vi "Plain Text.vi"(7 "Strip Line Ends? (F)":bool, 8 "error in (no error)":errorcluster, 11 "TermBuffer in":refnum<class "TermBuffer.lvclass">) -> (0 "error out":errorcluster, 2 "Contents":string, 3 "TermBuffer out":refnum<class "TermBuffer.lvclass">)   [LabVIEW 2020, in "Terminal.lvlib" / "TermBuffer.lvclass"]
uses:
  TermBuffer.lvclass
  TermBuffer.lvclass/TermBuffer.ctl
  TermLine/TermLine.lvclass
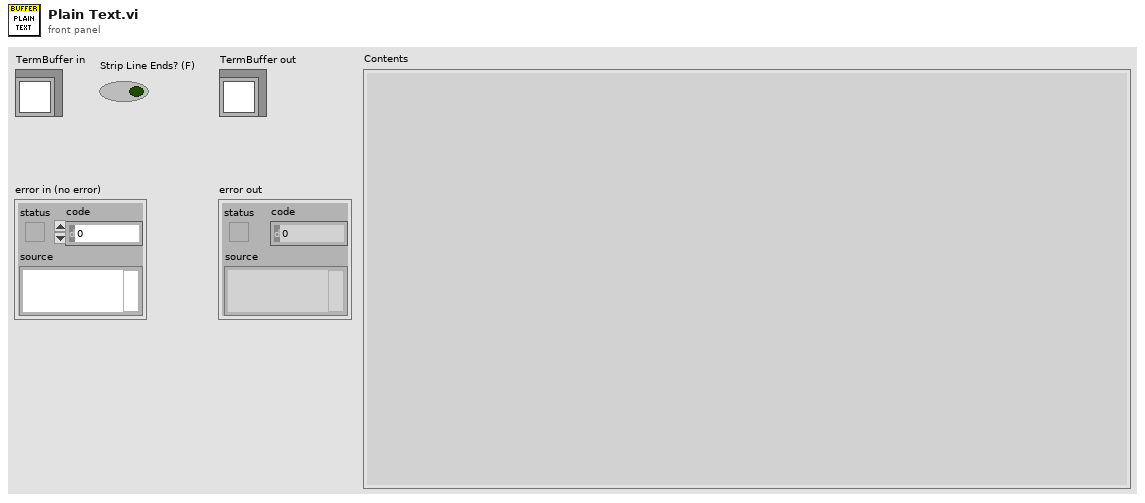
[diagram p1: front panel]
types:
  T1 = typedef "Terminal.lvlib/TermBuffer.lvclass/Ref Data.ctl" = cluster{"Lines":refnum<class "TermLine.lvclass">[], "Rows":i32, "Cols":i32}
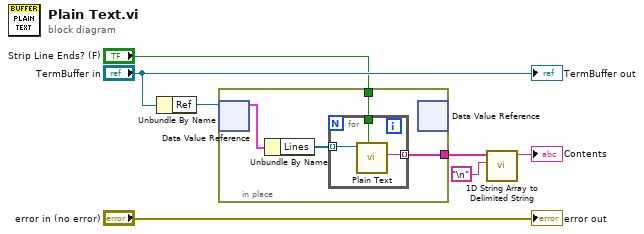
[diagram p0: block diagram]
diagram:
  n1 = Unbundle By Name("TermBuffer in") -> ("Ref"=w6:refnum<data-value>)
  n2 = in-place {
    in-place-border: [w9] -> w4
    in-place-border: "Strip Line Ends? (F)" -> [w8]
    n3 = in-place-dvr #1(w6) -> (w11:T1)  [unwired: 1 out]
    n4 = Unbundle By Name(w11) -> ("Lines"=w10:refnum<class "TermLine.lvclass">[])
    n5 = for {
      tunnel: w10 -> [w14] mode=indexing
      tunnel: [w13] -> w9 mode=indexing
      tunnel: w8 -> [w12]
      n6 = call "Plain Text.vi"("Strip End? (F)"=w12, "TermLine in"=w14) -> ("Line"=w13:string)  [unwired: 7 in, 2 out]
    }
    n7 = in-place-dvr #1() -> ()  [unwired: 1 in, 2 out]
  }
  n8 = call <vilib>:"1D String Array to Delimited String.vi"("delimiter"="\n", "string array"=w4) -> ("delimited string"=→"Contents":string)  [unwired: 9 in]
  "error out" <- "error in (no error)"
  "TermBuffer out" <- "TermBuffer in"
